vi "testWinkel.vi"(7 "Stopp":bool) -> (3 "Winkel":dbl format="%0.2f")   [LabVIEW 2014]
uses:
  <vilib>/Platform/TimedLoop/XDataNode/timing_clust.ctl
  <vilib>/Platform/TimedLoop/XDataNode/nitl_modes.ctl
  <vilib>/Platform/TimedLoop/XDataNode/wakeup.ctl
  <vilib>/DAQmx/read.llb/DAQmx Read (Counter DBL 1Chan 1Samp).vi
  <vilib>/DAQmx/miscellaneous.llb/DAQmx Fill In Error Info.vi
  <vilib>/Platform/TimedLoop/XDataNode/XDataNode.xnode
  <vilib>/Platform/TimedLoop/XDataNode/XDNodeRunTimeDep.lvlib
panel:
  out "1/s":dbl
  out "Signalverlaufsdiagramm":dbl(graph)
  out "Numerisch":i32
  out "frequency":dbl caption="Frequenz"
  out "data 2":dbl
  out "data":dbl format="%#.6f"
  out "Rundinstrument":dbl(knob) scale=-180.0..180.0
  out "error out":errorcluster caption="Fehler (Ausgang)"
  in  "error in":errorcluster caption="Fehler (Eingang)"
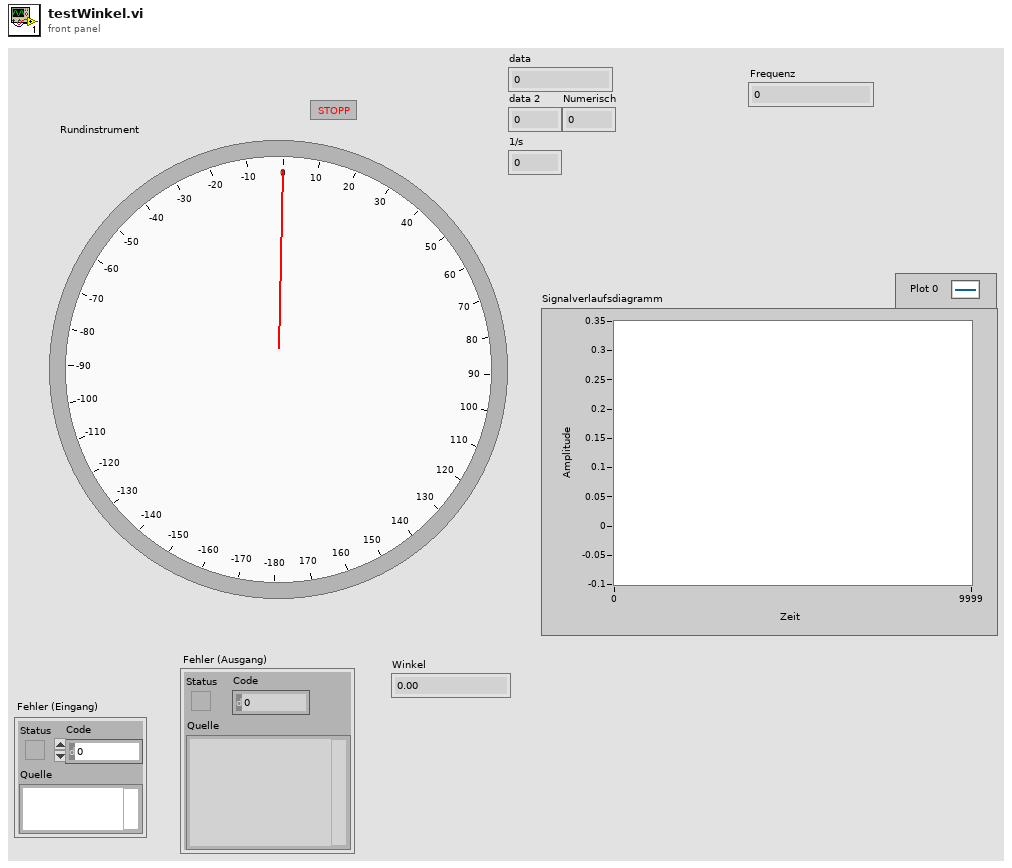
[diagram p1: front panel]
types:
  T1 = typedef "XDNodeRunTimeDep.lvlib/timing_clust.ctl" = cluster{"Expected End [f-1]":u64, "Actual End [f-1]":u64, "Finished Late? [f-1]":bool, "Expected End [i-1]":u64, "Actual End [i-1]":u64, "Finished Late? [i-1]":bool, "Expected Start [i]":u64, "Actual Start [i]":u64, "Expected Start [f]":u64, "Actual Start [f]":u64, "Source Name":string, "Structure Name":string, "Period":i64, "Deadline":i64, "Offset":i64, "Start":i64, "Priority":i32, "Timeout":i32, "Mode":T2, "Wakeup Reason":T3, "Error":errorcluster, "Source Type":string, "Secondary Source Type":string, "Global End Time":u64, "Global Start Time":u64, "Frame Duration":u64, "Iteration Duration":u64, "Assigned CPU":i32, "I/O Scan Engine Mode":u32}
  T2 = typedef "XDNodeRunTimeDep.lvlib/nitl_modes.ctl" = enum32{"No Change", "Process missed periods, maintain original phase", "Discard missed periods, maintain original phase", "Process missed periods, ignore original phase", "Discard missed periods, ignore original phase"}
  T3 = typedef "XDNodeRunTimeDep.lvlib/wakeup.ctl" = enum32{"Normal", "Aborted", "Asynchronous wakeup", "Timing source error", "Timed loop error", "Timeout"}
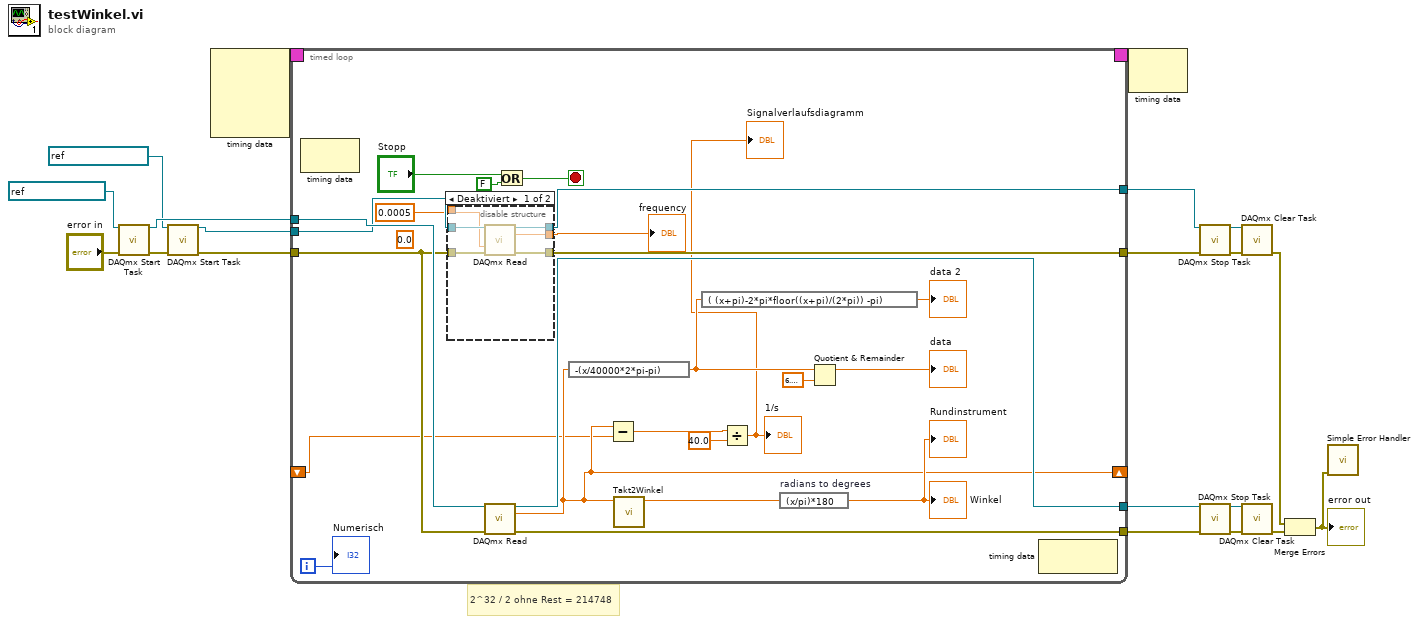
[diagram p0: block diagram]
diagram:
  # "2^32 / 2 ohne Rest = 214748"
  n1 = call <vilib>:"DAQmx Start Task.vi"("task/channels in"=refnum<k21> "Winkel1 Task", "error in"="error in") -> ("task out"=w16:refnum<k21>, "error out"=w3:errorcluster)  [unwired: 12 in]
  n2 = call <vilib>:"DAQmx Start Task.vi"("task/channels in"=refnum<k21> "FrequenzTask", "error in"=w3) -> ("task out"=w13:refnum<k21>, "error out"=w5:errorcluster)  [unwired: 12 in]
  n3 = node-c288() -> (w2:T1)  [unwired: 4 in]
  n4 = timed-loop {
    tunnel: w16 -> [w41]
    tunnel: [w40] -> w19
    tunnel: [w44] -> w20
    tunnel: w13 -> [w32]
    tunnel: [w31] -> w10
    tunnel: [w30] -> w7
    tunnel: w5 -> [w29]
    timing: w2 -> [_]
    timing-out: [_] -> w1
    shift-right: [w25] -> _
    shift-left: _ -> [w24]
    i -> [w28]
    stop <- w42 stop-if-true
    (unwired) 0.0 ("timeout")
    n5 = node-c288() -> ()  [unwired: 1 in, 1 out]
    n6 = disable-structure shown="Deaktiviert" {
      disable-tunnel: w32 -> [w50 _]
      disable-tunnel: [w49 _] -> w31
      disable-tunnel: [w48 _] -> w30
      disable-tunnel: w29 -> [w47 _]
      disable-tunnel: [w46 _] -> w27
      disable-tunnel: 0.0005 ("timeout") -> [w45 _]
      frame Disabled {
        n7 = call-poly <vilib>:"DAQmx Read.vi"("task/channels in"=w50, "timeout"=w45, "error in"=w47) -> ("task out"=w49:refnum<k21>, "data"=w46:dbl, "error out"=w48:errorcluster)  [unwired: 10 in]
      }
      frame Enabled {
      }
    }
    "frequency" <- w27
    n8 = call-poly <vilib>:"DAQmx Read.vi"("task/channels in"=w41, "error in"=w29) -> ("task out"=w44:refnum<k21>, "data"=w25:dbl, "error out"=w40:errorcluster)  [unwired: 11 in]
    n9 = Or(x="Stopp", y=FALSE) -> (x .or. y?=w42:bool)
    n10 = expression code="-(x/40000*2*pi-pi)"(w25) -> (w34:dbl)
    n11 = Subtract(x=w25, y=w24) -> (x-y=w23:dbl)
    n12 = call "Takt2Winkel.vi"("Taktzahl"=w25) -> ("Winkel (rad)"=w37:dbl)  [unwired: 10 in]
    n13 = expression code="( (x+pi)-2*pi*floor((x+pi)/(2*pi)) -pi)" ("Ausdrucksknoten")(w34) -> (→"data 2":dbl)
    n14 = Divide(x=w23, y=40.0) -> (x/y=→"Signalverlaufsdiagramm" →"1/s":dbl)
    n15 = expression code="(x/pi)*180" "radians to degrees"(w37) -> (→"Winkel" →"Rundinstrument":dbl)
    n16 = Quotient & Remainder(x=w34, y=6.283185307179586) -> (x-y*floor(x/y)=→"data":dbl)  [unwired: 1 out]
    n17 = node-c288() -> ()  [unwired: 1 in, 1 out]
    "Numerisch" <- w28
  }
  n18 = node-c288(w1) -> ()  [unwired: 1 out]
  n19 = call <vilib>:"DAQmx Stop Task.vi"("task/channels in"=w10, "error in"=w7) -> ("task out"=w12:refnum<k21>, "error out"=w11:errorcluster)  [unwired: 12 in]
  n20 = call <vilib>:"DAQmx Stop Task.vi"("task/channels in"=w20, "error in"=w19) -> ("task out"=w18:refnum<k21>, "error out"=w17:errorcluster)  [unwired: 12 in]
  n21 = call <vilib>:"DAQmx Clear Task.vi"("task in"=w12, "error in"=w11) -> ("error out"=w8:errorcluster)  [unwired: 13 in]
  n22 = call <vilib>:"DAQmx Clear Task.vi"("task in"=w18, "error in"=w17) -> ("error out"=w9:errorcluster)  [unwired: 13 in]
  n23 = Merge Errors(w8, w9) -> (w6:errorcluster)
  "error out" <- w6
  n24 = call <vilib>:"Simple Error Handler.vi"("error in (no error)"=w6) -> ()  [unwired: 4 in, 5 out]
